vi "CRC16校验.vi"(10 "输入数据_U16":u16[](array[numeric])) -> (1 "低字节":u8 format="%x", 3 "高字节":u8 format="%x")   [LabVIEW 2010]
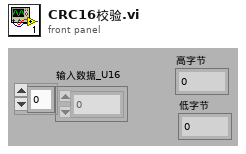
[diagram p1: front panel]
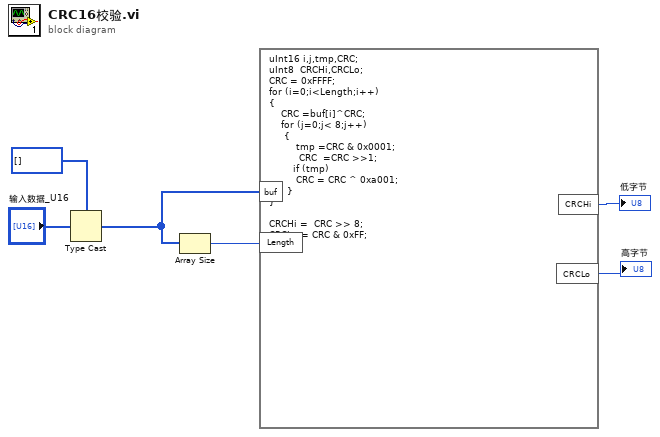
[diagram p0: block diagram]
diagram:
  n1 = Type Cast(type=u8[] [], x="输入数据_U16") -> (*(type *) &x=w1:u8[])
  n2 = Array Size(array=w1) -> (size(s)=w4:i32)
  n3 = formula code="uInt16 i,j,tmp,CRC;\nuInt8  CRCHi,CRCLo;\nCRC = 0xFFFF;\nfor (i=0;i<Length;i++)\n{\n    CRC =buf[i]^CRC;\n    for (j=0;j< 8;j++)\n     {\n         tmp =CRC & 0x0001;\n          CRC  =CRC >>1;\n        if (tmp)\n         CRC = CRC ^ 0xa001;    \n      }\n}\n\nCRCHi =  CRC >> 8;\nCRCLo = CRC & 0xFF;"("buf"=w1, "Length"=w4) -> ("CRCLo"=→"高字节":u8, "CRCHi"=→"低字节":u8)
